vi "Clear Specific Error.vi"(5 "clear any warning (F)":bool, 7 "clear any error (F)":bool, 8 "error in (no error)":errorcluster, 11 "code":i32) -> (0 "error out":errorcluster, 2 "cleared?":bool, 3 "code found?":bool)   [LabVIEW 2017, in "NI_Robotics Utilities.lvlib"]
uses:
  <vilib>/robotics/Utilities/NI_Robotics Utilities.lvlib
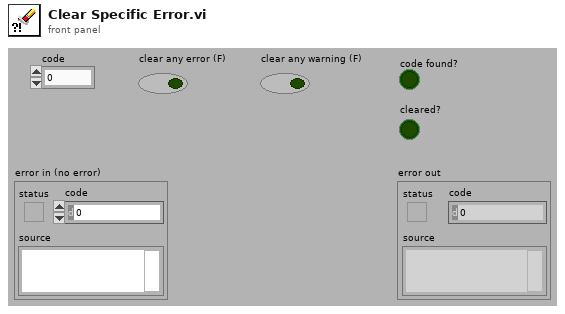
[diagram p1: front panel]
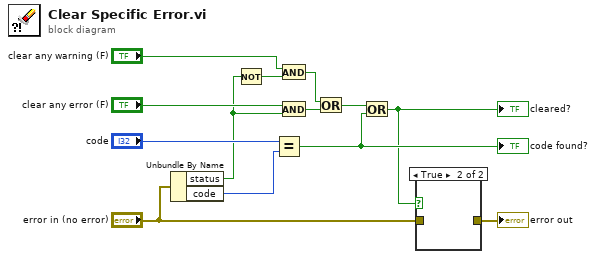
[diagram p0: block diagram]
diagram:
  n1 = Unbundle By Name("error in (no error)") -> ("status"=w10:bool, "code"=w13:i32)
  n2 = Not(x=w10) -> (.not. x?=w9:bool)
  n3 = Equal?(x="code", y=w13) -> (x = y?=w4:bool)
  "code found?" <- w4
  n4 = And(x="clear any warning (F)", y=w9) -> (x .and. y?=w6:bool)
  n5 = And(x="clear any error (F)", y=w10) -> (x .and. y?=w7:bool)
  n6 = Or(x=w6, y=w7) -> (x .or. y?=w5:bool)
  n7 = Or(x=w5, y=w4) -> (x .or. y?=w2:bool)
  "cleared?" <- w2
  n8 = case shown="True" w2 {
    tunnel: "error in (no error)" -> [w14 _]
    tunnel: [w14 _] -> w1
    frame False {
    }
    frame True {
    }
  }
  "error out" <- w1
